vi "Find PID in Configuration.vi"(10 "PID Loop ID in":string, 11 "Tagbus PID Module configuration in":refnum<class "PID Module configuration.lvclass">) -> (2 "index":i32, 3 "Tagbus PID Module configuration out":refnum<class "PID Module configuration.lvclass">)   [LabVIEW 2013, in "PID Module configuration.lvclass"]
doc: "This VI locates a given PID Loop in the Module Configuration and returns it's index if found, or -1 if not found."
uses:
  PID Module configuration.lvclass
  PID Module configuration.lvclass/PID Module configuration.ctl
  PID Loop/PID Loop.lvclass
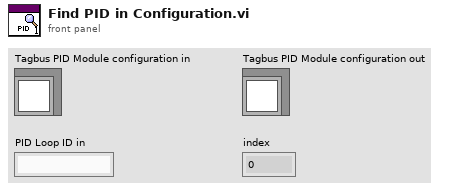
[diagram p1: front panel]
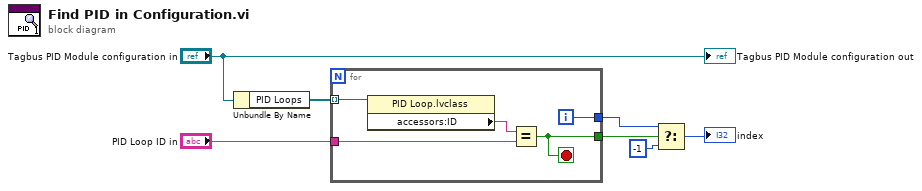
[diagram p0: block diagram]
diagram:
  n1 = Unbundle By Name("Tagbus PID Module configuration in") -> ("PID Loops"=w3:refnum<class "PID Loop.lvclass">[])
  n2 = for {
    tunnel: [w12] -> w5
    tunnel: [w11] -> w6
    tunnel: w3 -> [w10] mode=indexing
    tunnel: "PID Loop ID in" -> [w8]
    i -> [w12]
    stop <- w11 stop-if-true
    n3 = property class="PID Loop.lvclass"(reference=w10) -> ("accessors:ID"=w9:string)  [unwired: 1 in, 2 out]
    n4 = Equal?(x=w9, y=w8) -> (x = y?=w11:bool)
  }
  n5 = Select(t=w5, s=w6, f=-1) -> (s? t:f=→"index":i32)
  "Tagbus PID Module configuration out" <- "Tagbus PID Module configuration in"
